vi "Analysis.AddedItem.vi"(8 "error in (no error)":errorcluster, 10 "property names":string[](array[string]), 11 "property values":variant[](array[variant])) -> (0 "error out":errorcluster, 2 "Result?":bool, 3 "Variant out":variant)   [LabVIEW 2015, in "Analysis.lvlib"]
uses:
  Analysis.lvlib
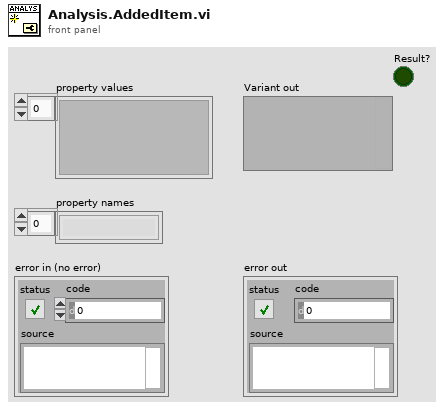
[diagram p1: front panel]
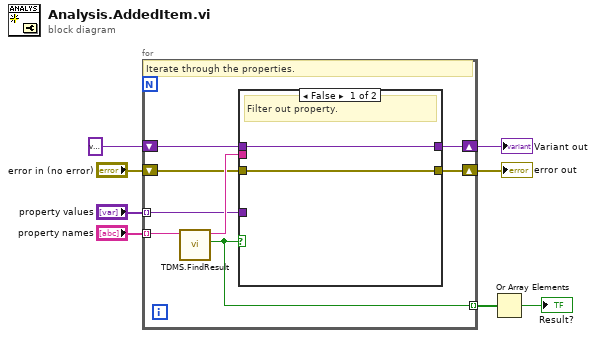
[diagram p0: block diagram]
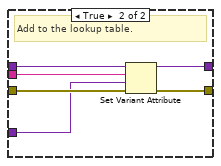
[diagram p2: hidden frame]
diagram:
  n1 = for {
    shift-right: [w15] -> w4
    shift-left: variant ("Variant in") -> [w16]
    tunnel: "property names" -> [w14] mode=indexing
    tunnel: "property values" -> [w12] mode=indexing
    shift-right: [w11] -> w8
    shift-left: "error in (no error)" -> [w10]
    tunnel: [w9] -> w2 mode=indexing
    # "Iterate through the properties."
    n2 = call "TDMS.FindResult.vi"("Property in"=w14) -> ("Result"=w9:bool, "Property out"=w13:string)  [unwired: 8 in, 1 out]
    n3 = case shown="False" w9 {
      tunnel: w16 -> [w18 w24]
      tunnel: [w18 w23] -> w15
      tunnel: w13 -> [_ w22]
      tunnel: w12 -> [_ w19]
      tunnel: [w17 w21] -> w11
      tunnel: w10 -> [w17 w20]
      frame False {
        # "Filter out property."
      }
      frame True {
        # "Add to the lookup table."
        n4 = Set Variant Attribute(Variant=w24, name=w22, value=w19, error in=w20) -> (Variant out=w23:variant, error out=w21:errorcluster)  [unwired: 1 out]
      }
    }
  }
  "error out" <- w8
  "Variant out" <- w4
  n5 = Or Array Elements(Boolean array=w2) -> (logical OR=→"Result?":bool)
